vi "sub_plot_beamCurrent_and_trip_events.vi"(9 "要看前幾個小時":dbl=12.0 format="%#_13g", 10 "最新時間":dbl format="%#_13g", 11 "T:Slow\nF:Fast":bool) -> (0 "Y min value":dbl, 1 "Y max value":dbl, 2 "X min value":dbl, 3 "X max value":dbl, 4 "BeamCurrent History":cluster{dbl[], dbl[]}[](graph), 6 "result":string)   [LabVIEW 2017]
uses:
  <vilib>/addons/database/Connection.llb/DB Tools Open Connec (Path).vi
  <vilib>/addons/database/Connection.llb/Conn Execute.vi
  <vilib>/addons/database/Recordset.llb/Rec Fetch Recordset Data (R).vi
  <vilib>/addons/database/Recordset.llb/Rec Destroy - Connection.vi
  <vilib>/addons/database/_DB Variant To Data/Database Variant To Data.xnode
  <vilib>/addons/database/NI_Database_API.lvlib
panel:
  out "error out 4":errorcluster
  # "如果目前系統在down time 尚未恢復，就會以-----時間當作resume time"
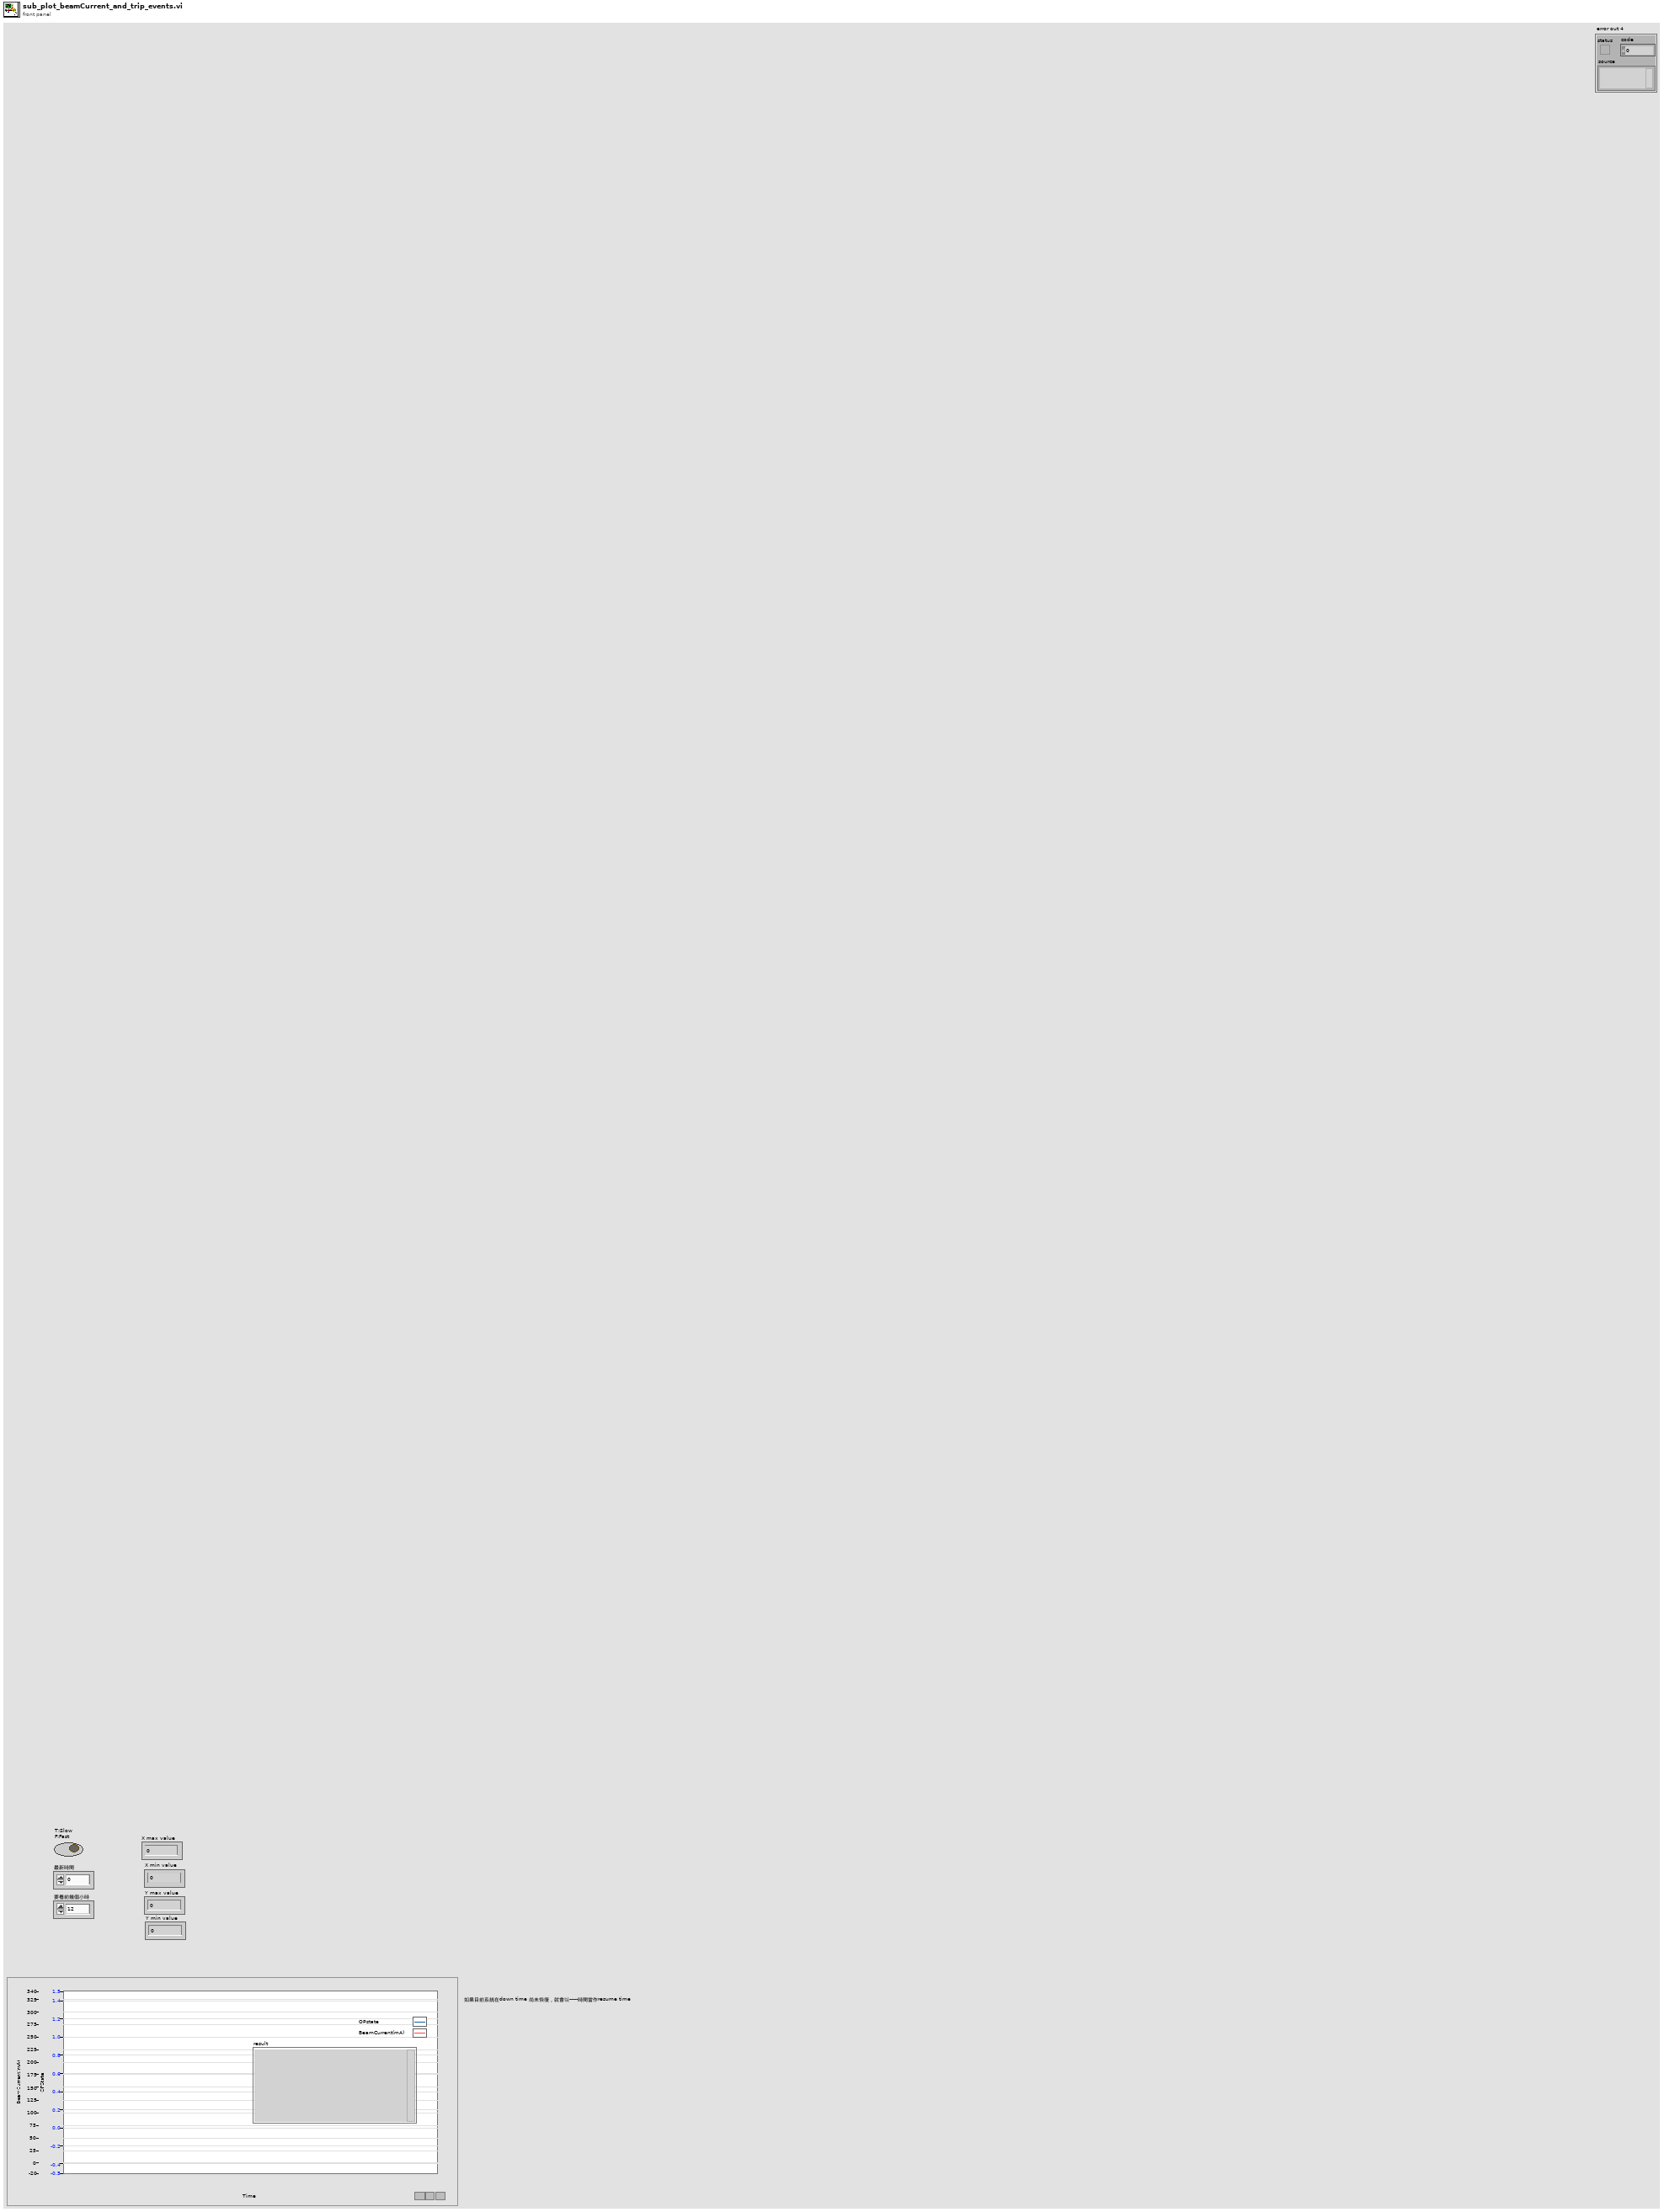
[diagram p1: front panel]
types:
  T1 = typedef "NI_Database_API.lvlib/Conn ObjectReference.ctl" = refnum<k1>
  T2 = typedef "NI_Database_API.lvlib/Rec ObjectReference.ctl" = refnum<k1>
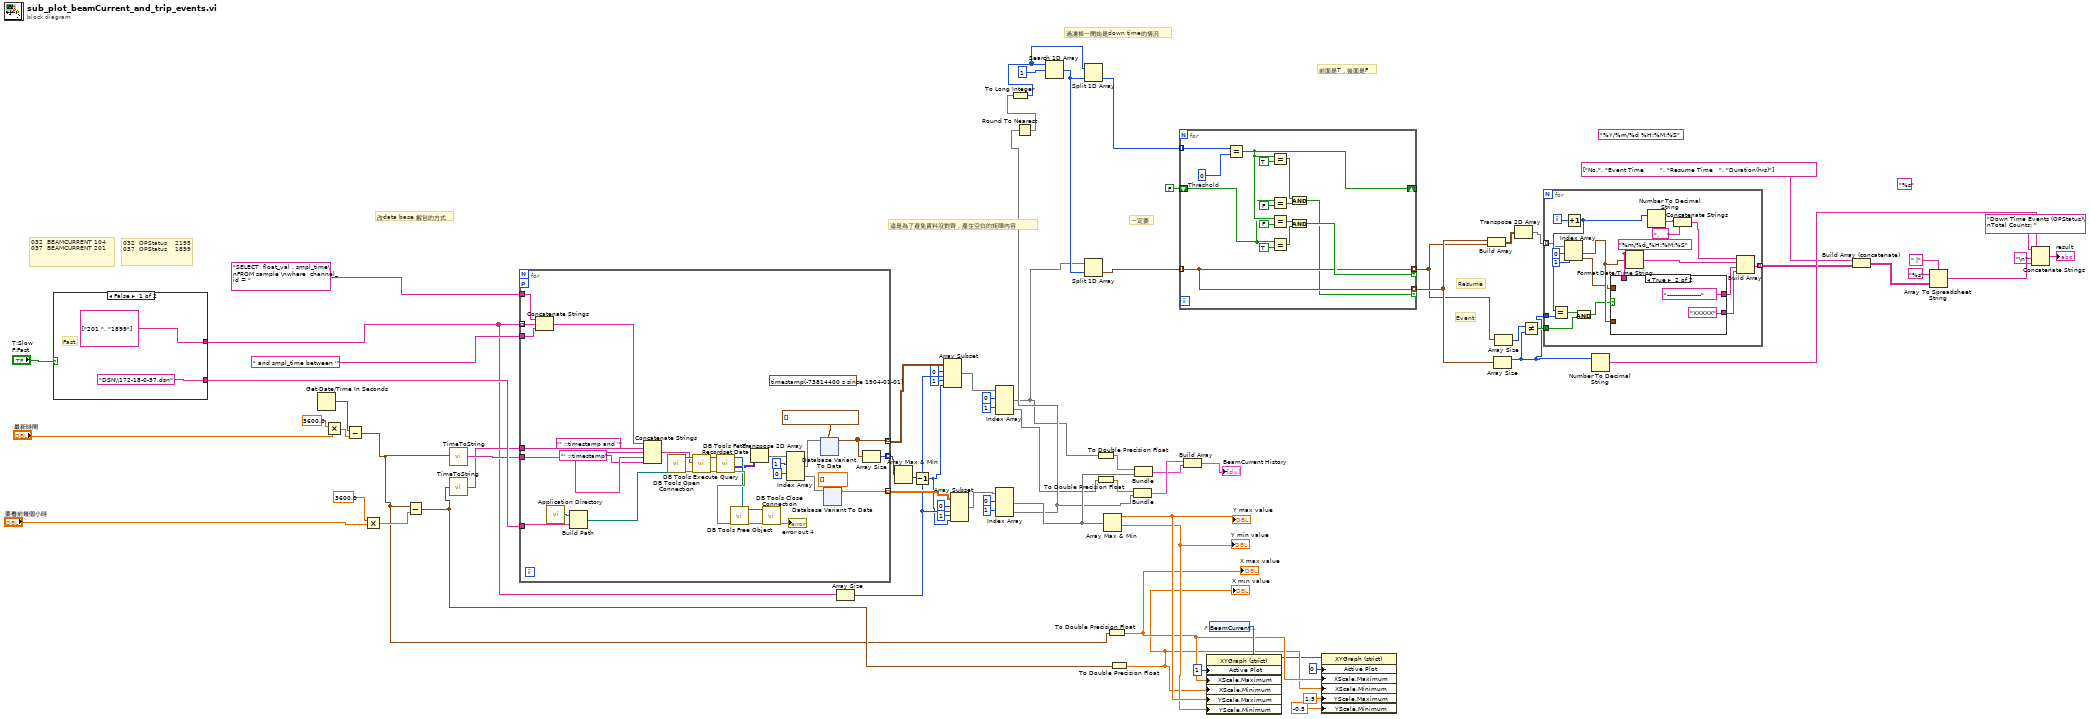
[diagram p0: block diagram]
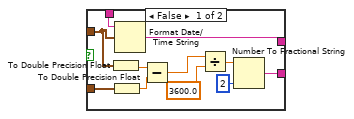
[diagram p2: hidden frame]
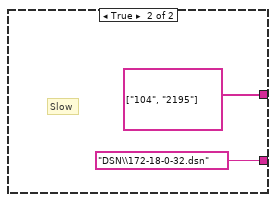
[diagram p3: hidden frame]
diagram:
  (unwired) "%s" ("format string")
  (unwired) "%Y/%m/%d %H:%M:%S" ("time format string (%c)")
  # "Resume"
  # "Event"
  # "一定要"
  # "這是為了避免資料沒對齊，產生空白的矩陣內容"
  # "前面是T，後面是F"
  # "過濾掉一開始是down time的情況"
  # "032  OPStatus    2195\n037  OPStatus    1899"
  # "032  BEAMCURRENT 104\n037  BEAMCURRENT 201"
  # "改data base 解包的方式"
  n1 = case shown="False" "T:Slow\nF:Fast" {
    tunnel: ["DSN\\172-18-0-37.dsn" "DSN\\172-18-0-32.dsn"] -> w75
    tunnel: [string[] ["201 ", "1899"] string[] ["104", "2195"]] -> w34
    frame False {
      # "Fast"
    }
    frame True {
      # "Slow"
    }
  }
  n2 = Get Date/Time In Seconds() -> (seconds since 1Jan1904=w40:timestamp)
  n3 = Multiply(x=3600.0 ("y"), y="最新時間") -> (x*y=w42:dbl)
  n4 = Subtract(x=w40, y=w42) -> (x-y=w39:timestamp)
  n5 = Multiply(x=3600.0 ("y"), y="要看前幾個小時") -> (x*y=w72:dbl)
  n6 = Subtract(x=w39, y=w72) -> (x-y=w50:timestamp)
  n7 = call "TimeToString.vi"("Time Stamp Control"=w39) -> ("result string"=w74:string)
  n8 = call "TimeToString.vi"("Time Stamp Control"=w50) -> ("result string"=w73:string)
  n9 = for {
    tunnel: w75 -> [w108]
    tunnel: w74 -> [w106]
    tunnel: w73 -> [w105]
    tunnel: "SELECT  float_val , smpl_time\nFROM sample \nwhere  channel_id = " ("result string") -> [w86]
    tunnel: w34 -> [w85] mode=indexing
    tunnel: " and smpl_time between '" ("result string") -> [w84]
    workers-P: _ -> [_]
    tunnel: [w81] -> w38 mode=indexing
    tunnel: [w82] -> w35 mode=indexing
    tunnel: [w80] -> w30 mode=indexing
    (unwired) timestamp(-73814400 s since 1904-01-01)
    n10 = Concatenate Strings(w86, w85, w84) -> (w83:string)
    n11 = call <vilib>:"Application Directory.vi"() -> ("Application Directory"=w107:path)
    n12 = Build Path(base path=w107, name or relative path=w108) -> (appended path=w109:path)
    n13 = Concatenate Strings(w83, w105, "' ::timestamp and '" ("result string"), w106, "' ::timestamp" ("result string")) -> (w95:string)
    n14 = call-poly <vilib>:"DB Tools Open Connection.vi"("connection information"=w109) -> ("error out"=w104:errorcluster, "connection reference"=w103:T1)  [unwired: 7 in]
    n15 = call-poly <vilib>:"DB Tools Execute Query.vi"("error in (no error)"=w104, "SQL query"=w95, "connection reference"=w103) -> ("error out"=w101:errorcluster, "recordset reference"=w102:T2)  [unwired: 5 in]
    n16 = call-poly <vilib>:"DB Tools Fetch Recordset Data.vi"("error in (no error)"=w101, "recordset reference"=w102) -> ("error out"=w111:errorcluster, "recordset data"=w94:variant[][], "recordset reference out"=w100:T2)  [unwired: 3 in]
    n17 = call-poly <vilib>:"DB Tools Free Object.vi"("error in (no error)"=w111, "recordset reference"=w100) -> ("error out"=w98:errorcluster, "connection reference"=w99:T1)  [unwired: 8 in]
    n18 = Transpose 2D Array(2D array=w94) -> (transposed array=w91:variant[][])
    n19 = call <vilib>:"DB Tools Close Connection.vi"("error in (no error)"=w98, "connection reference"=w99) -> ("error out"=→"error out 4":errorcluster)  [unwired: 5 in]
    n20 = Index Array(array=w91, index (row) #1=1 ("index (row)"), index (row) #2=0 ("index (row)")) -> (element #1=w89:variant[], element #2=w88:variant[])  [unwired: 2 in]
    n21 = xnode "Database Variant To Data"("database variant"=w89, "type"=timestamp[] []) -> ("data"=w81:timestamp[])  [unwired: 1 in, 1 out]
    n22 = xnode "Database Variant To Data"("database variant"=w88, "type"=dbl[] []) -> ("data"=w82:dbl[])  [unwired: 1 in, 1 out]
    n23 = Array Size(array=w81) -> (size(s)=w80:i32)
  }
  n24 = Array Size(array=w34) -> (size(s)=w33:i32)
  n25 = Array Max & Min(array=w30) -> (min value=w29:i32)  [unwired: 3 out]
  n26 = Decrement(x=w29) -> (x-1=w28:i32)
  n27 = Array Subset(array=w38, index (row)=0 ("index"), length (row)=w33, index (col)=1 ("index"), length (col)=w28) -> (w27:timestamp[][])
  n28 = Array Subset(array=w35, index (row)=0 ("index"), length (row)=w33, index (col)=1 ("index"), length (col)=w28) -> (w26:dbl[][])
  n29 = Index Array(array=w27, index (row) #1=0 ("index (row)"), index (row) #2=1 ("index (row)")) -> (element #1=w4:timestamp[], element #2=w2:timestamp[])  [unwired: 2 in]
  n30 = Index Array(array=w26, index (row) #1=0 ("index (row)"), index (row) #2=1 ("index (row)")) -> (element #1=w51:dbl[], element #2=w13:dbl[])  [unwired: 2 in]
  n31 = Round To Nearest(number=w13) -> (nearest integer value=w12:dbl[])
  n32 = To Long Integer(number=w12) -> (32bit integer=w11:i32[])
  n33 = Search 1D Array(1D array=w11, element=1) -> (index of element=w45:i32)  [unwired: 1 in]
  n34 = Split 1D Array(array=w11, index=w45) -> (second subarray=w46:i32[])  [unwired: 1 out]
  n35 = Split 1D Array(array=w4, index=w45) -> (second subarray=w44:timestamp[])  [unwired: 1 out]
  n36 = To Double Precision Float(number=w4) -> (double precision float=w3:dbl[])
  n37 = To Double Precision Float(number=w2) -> (double precision float=w1:dbl[])
  n38 = Array Max & Min(array=w51) -> (max value=w55:dbl, min value=w54:dbl)  [unwired: 2 out]
  "Y max value" <- w55
  "Y min value" <- w54
  n39 = To Double Precision Float(number=w39) -> (double precision float=w20:dbl)
  "X max value" <- w20
  n40 = To Double Precision Float(number=w50) -> (double precision float=w19:dbl)
  "X min value" <- w19
  n41 = Bundle(w1, w13) -> (w24:cluster{dbl[], dbl[]})  [unwired: 1 in]
  n42 = Bundle(w3, w51) -> (w23:cluster{dbl[], dbl[]})  [unwired: 1 in]
  n43 = for {
    tunnel: w46 -> [w216] mode=indexing
    shift-right: [w214] -> _
    shift-left: FALSE -> [w213]
    tunnel: w44 -> [w203] mode=indexing
    tunnel: [w203] -> w7 mode=indexing if=w204
    tunnel: [w203] -> w9 mode=indexing if=w202
    w215 = 0  # Threshold
    n44 = Equal?(x=w216, y=w215) -> (x = y?=w214:bool)
    n45 = Equal?(x=w214, y=TRUE) -> (x = y?=w206:bool)
    n46 = Equal?(x=w213, y=FALSE) -> (x = y?=w205:bool)
    n47 = Equal?(x=w214, y=FALSE) -> (x = y?=w210:bool)
    n48 = Equal?(x=w213, y=TRUE) -> (x = y?=w209:bool)
    n49 = And(x=w206, y=w205) -> (x .and. y?=w202:bool)
    n50 = And(x=w210, y=w209) -> (x .and. y?=w204:bool)
  }
  n51 = Build Array(w24, w23) -> (→"BeamCurrent History":cluster{dbl[], dbl[]}[])
  n52 = control-ref of="BeamCurrent History"() -> (w56:refnum<vi>)
  n53 = property on="Property Node" class="XYGraph (strict)"(reference=w56, "Active Plot"=u32 1, "XScale.Maximum"=w20, "XScale.Minimum"=w19, "YScale.Maximum"=w55, "YScale.Minimum"=w54) -> (reference out=w16:refnum<vi>)  [unwired: 1 in, 1 out]
  n54 = property on="Property Node" class="XYGraph (strict)"(reference=w16, "Active Plot"=u32 0, "XScale.Maximum"=w20, "XScale.Minimum"=w19, "YScale.Maximum"=1.5 ("Y Scale.Range:Maximum"), "YScale.Minimum"=-0.5 ("Y Scale.Range:Minimum")) -> ()  [unwired: 1 in, 2 out]
  n55 = Build Array(w9, w7) -> (w6:timestamp[][])
  n56 = Array Size(array=w9) -> (size(s)=w10:i32)
  n57 = Array Size(array=w7) -> (size(s)=w14:i32)
  n58 = Transpose 2D Array(2D array=w6) -> (transposed array=w5:timestamp[][])
  n59 = Not Equal?(x=w14, y=w10) -> (x != y?=w15:bool)
  n60 = for {
    tunnel: [w234] -> w57 mode=indexing
    tunnel: w15 -> [w226]
    tunnel: w10 -> [w227]
    tunnel: w5 -> [w222] mode=indexing
    i -> [w225]
    w230 = "%m/%d_%H:%M:%S" ("time format string (%c)")
    n61 = Index Array(array=w222, index #1=0 ("index"), index #2=1 ("index")) -> (element #1=w220:timestamp, element #2=w218:timestamp)
    n62 = Increment(x=w225) -> (x+1=w224:i32)
    n63 = Equal?(x=w224, y=w227) -> (x = y?=w223:bool)
    n64 = And(x=w223, y=w226) -> (x .and. y?=w217:bool)
    n65 = case shown="True" w217 {
      tunnel: w230 -> [w246 _]
      tunnel: [w245 "-----------------" ("date/time string")] -> w229
      tunnel: w218 -> [w244 _]
      tunnel: w220 -> [w243 _]
      tunnel: [w236 "XXXXX"] -> w228
      frame False {
        n66 = To Double Precision Float(number=w244) -> (double precision float=w241:dbl)
        n67 = To Double Precision Float(number=w243) -> (double precision float=w242:dbl)
        n68 = Format Date/Time String(time format string (%c)=w246, seconds (now)=w244) -> (date/time string=w245:string)  [unwired: 1 in]
        n69 = Subtract(x=w241, y=w242) -> (x-y=w240:dbl)
        n70 = Divide(x=w240, y=3600.0) -> (x/y=w238:dbl)
        n71 = Number To Fractional String(number=w238, precision (6)=i16 2) -> (F-format string=w236:string)  [unwired: 2 in]
      }
      frame True {
      }
    }
    n72 = Format Date/Time String(time format string (%c)=w230, seconds (now)=w220) -> (date/time string=w235:string)  [unwired: 1 in]
    n73 = Number To Decimal String(number=w224) -> (decimal integer string=w233:string)  [unwired: 1 in]
    n74 = Concatenate Strings(w233, ".    " ("string")) -> (w231:string)
    n75 = Build Array(w231, w235, w229, w228) -> (w234:string[])
  }
  n76 = Number To Decimal String(number=w10) -> (decimal integer string=w63:string)  [unwired: 1 in]
  n77 = Build Array (concatenate)(string[] ["No.", "Event Time        ", "Resume Time   ", "Duration(hrs)"], w57) -> (w61:string[][])
  n78 = Array To Spreadsheet String(delimiter (Tab)=" |", array=w61, 3:"%s" ("format string")) -> (spreadsheet string=w65:string)
  n79 = Concatenate Strings("Down Time Events (OPStatus)\nTotal Counts: ", w63, "\n" ("string"), w65) -> (→"result":string)
